vi "DELETE ESCALATION.vi"(8 "error in (no error)":errorcluster, 11 "connection reference":T1) -> (0 "error out":errorcluster, 3 "connection reference out":T1)   [LabVIEW 2017]
uses:
  <vilib>/addons/database/Connection.llb/Conn ObjectReference.ctl
  <vilib>/addons/database/Connection.llb/DB Tools Open Connec (Path).vi
  <vilib>/addons/database/NI_Database_API.lvlib
panel:
  in  "CANCEL":bool
  in  "Select Serial Number":string(combo)
  in  "DELETE":bool
  # "Delete Escalation Detail"
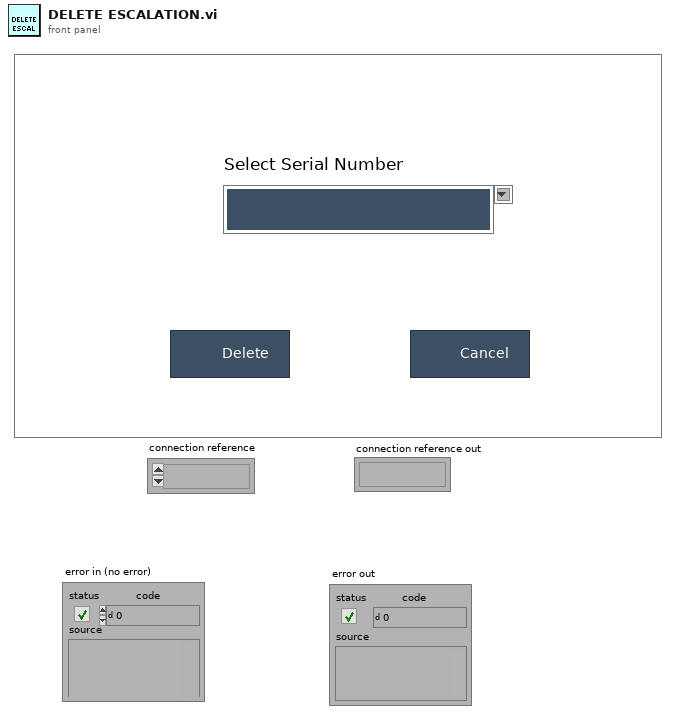
[diagram p1: front panel]
types:
  T1 = typedef "NI_Database_API.lvlib/Conn ObjectReference.ctl" = refnum<k1>
  T2 = enum32{"invalid app kind", "Development System", "Run Time System", "Student Edition", "Embedded LabVIEW", "Evaluation", "Custom"}
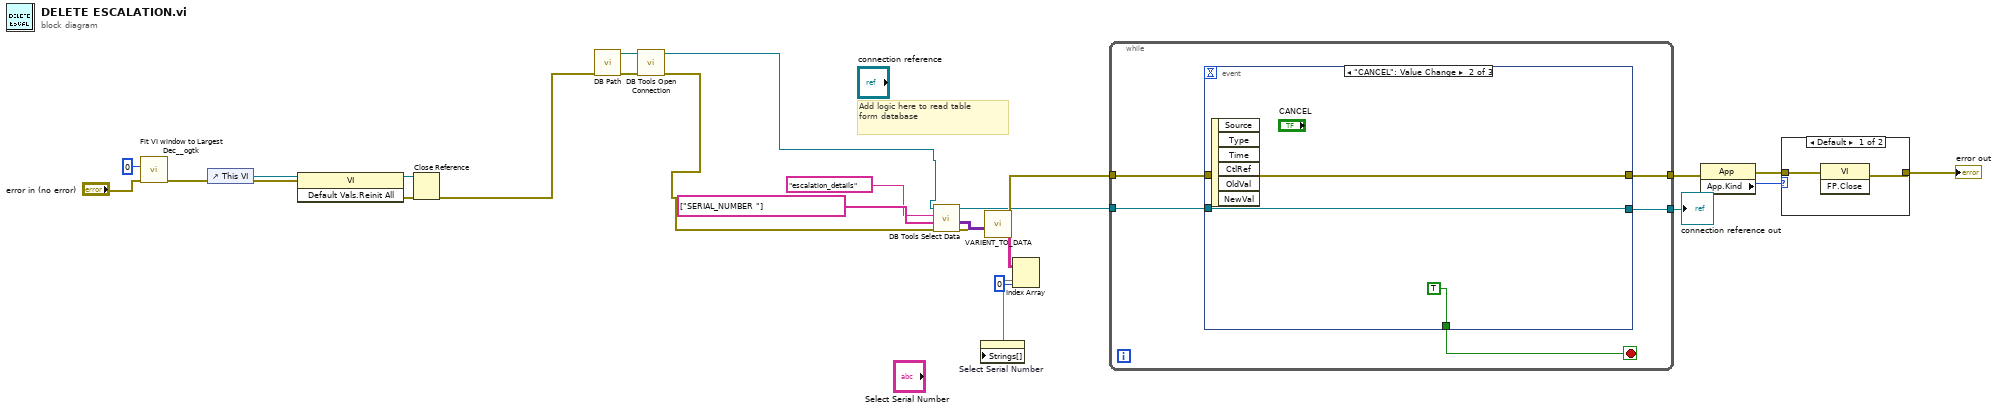
[diagram p0: block diagram]
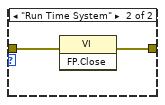
[diagram p2: hidden frame]
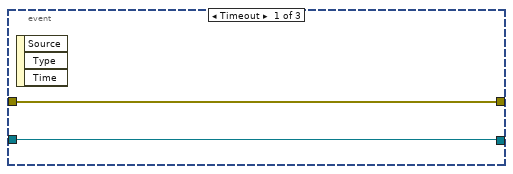
[diagram p3: hidden frame]
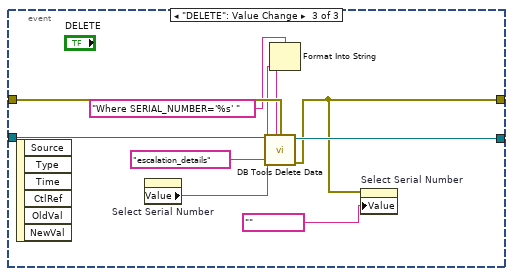
[diagram p4: hidden frame]
diagram:
  # "Add logic here to read table\nform database"
  n1 = call <userlib>:"Fit VI window to Largest Dec__ogtk.vi"("error in (no error)"="error in (no error)", "border spacing (2 px)"=0) -> ("error out"=w7:errorcluster)  [unwired: 4 in, 1 out]
  n2 = control-ref of="This VI"() -> (w25:refnum<vi>)
  n3 = invoke class="VI" method="Default Vals.Reinit All"(reference=w25, error in=w7) -> (reference out=w23:refnum<vi>, error out=w24:errorcluster)  [unwired: 1 in, 1 out]
  n4 = Close Reference(reference=w23, error in (no error)=w24) -> (error out=w3:errorcluster)
  n5 = call "DB Path.vi"("error in"=w3) -> ("error out"=w5:errorcluster, "DB Path"=w4:path)  [unwired: 9 in]
  n6 = call-poly <vilib>:"DB Tools Open Connection.vi"("error in (no error)"=w5, "connection information"=w4) -> ("error out"=w2:errorcluster, "connection reference"=w1:T1)  [unwired: 6 in]
  n7 = call <vilib>:"DB Tools Select Data.vi"("error in (no error)"=w2, "columns"=string[] ["SERIAL_NUMBER "], "table"="escalation_details", "connection reference"=w1) -> ("error out"=w17:errorcluster, "data"=w18:variant[][], "connection reference out"=w10:T1)  [unwired: 2 in]
  n8 = call "VARIENT_TO_DATA.vi"("data"=w18, "error in (no error)"=w17) -> ("Table"=w13:string[][], "error out"=w14:errorcluster)  [unwired: 7 in]
  n9 = Index Array(array=w13, index (col)=0 ("disabled index (col)")) -> (element=w11:string[])  [unwired: 1 in]
  n10 = property on="Select Serial Number" class="CmbBox"("Strings[]"=w11) -> ()  [unwired: 2 in, 2 out]
  n11 = while {
    tunnel: w14 -> [w30]
    tunnel: [w29] -> w19
    tunnel: w10 -> [w28]
    tunnel: [w27] -> w9
    stop <- w26 stop-if-true
    n12 = event shown="[1] \"CANCEL\": Value Change" {
      selector: _ -> [_ _ _]
      dyn-events: _ -> [_ _ _]
      timeout: _ -> [_ _ _]
      tunnel: w30 -> [w32 w33 w43]
      tunnel: [w32 w33 w36] -> w29
      tunnel: w28 -> [w31 w34 w44]
      tunnel: [w31 w34 w42] -> w27
      tunnel: [_ TRUE _] -> w26
      event Timeout {
        n13 = event-data() -> ()  [unwired: 1 in, 3 out]
      }
      event "CANCEL": Value Change {
        n14 = event-data() -> ()  [unwired: 1 in, 6 out]
      }
      event "DELETE": Value Change {
        n15 = event-data() -> ()  [unwired: 1 in, 6 out]
        n16 = property on="Select Serial Number" class="CmbBox"() -> ("Value"=w40:string)  [unwired: 2 in, 2 out]
        n17 = Format Into String(format string="Where SERIAL_NUMBER='%s' " ("condition"), w40) -> (resulting string=w39:string)  [unwired: 2 in, 1 out]
        n18 = call <vilib>:"DB Tools Delete Data.vi"("condition"=w39, "error in (no error)"=w43, "table"="escalation_details", "connection reference"=w44) -> ("error out"=w36:errorcluster, "connection reference out"=w42:T1)  [unwired: 6 in]
        n19 = property on="Select Serial Number" class="CmbBox"(error in=w36, "Value"="") -> ()  [unwired: 1 in, 2 out]
      }
    }
  }
  "connection reference out" <- w9
  n20 = property class="App"(error in=w19) -> (error out=w21:errorcluster, "App.Kind"=w22:T2)  [unwired: 1 in, 1 out]
  n21 = case shown="Default" w22 {
    tunnel: w21 -> [w46 w48]
    tunnel: [w45 w47] -> w20
    frame Default {
      n22 = invoke class="VI" method="FP.Close"(error in=w46) -> (error out=w45:errorcluster)  [unwired: 2 in, 2 out]
    }
    frame "Run Time System" {
      n23 = invoke class="VI" method="FP.Close"(error in=w48) -> (error out=w47:errorcluster)  [unwired: 2 in, 2 out]
    }
  }
  "error out" <- w20
